vi "字符串至进制转换（个人编写）.vi"(1 "字符串":string) -> (0 "十六进制字符串":string)   [LabVIEW 2012]
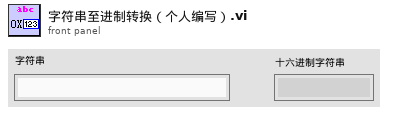
[diagram p1: front panel]
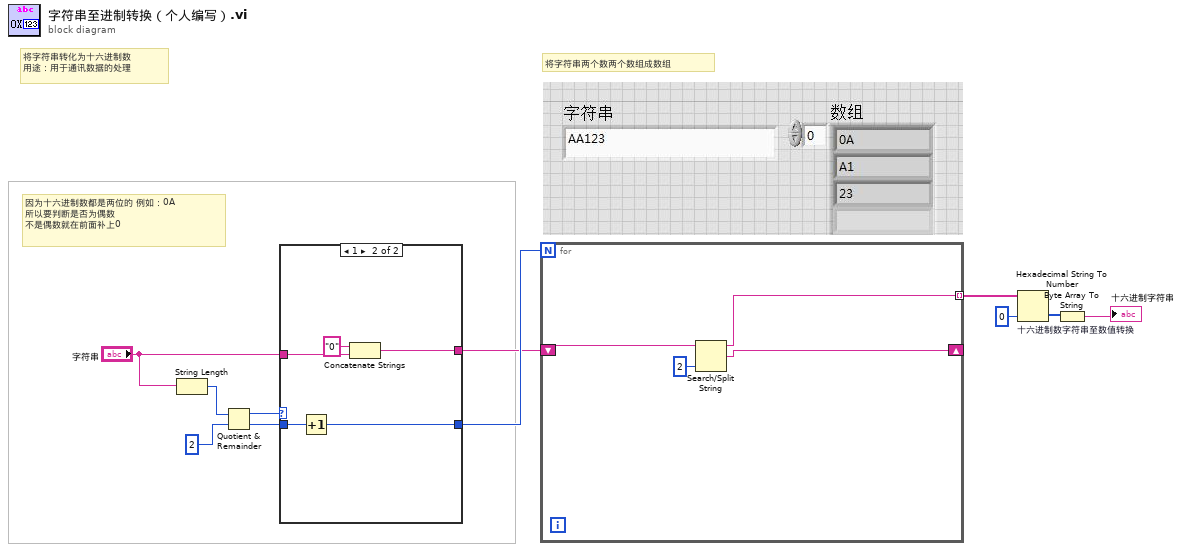
[diagram p0: block diagram]
diagram:
  # "将字符串转化为十六进制数\n用途：用于通讯数据的处理"
  # "将字符串两个数两个数组成数组"
  # "因为十六进制数都是两位的 例如：0A\n所以要判断是否为偶数\n不是偶数就在前面补上0"
  n1 = String Length(string="字符串") -> (length=w8:i32)
  n2 = Quotient & Remainder(x=w8, y=2) -> (x-y*floor(x/y)=w10:i32, floor(x/y)=w7:i32)
  n3 = case shown="1" w10 {
    tunnel: "字符串" -> [w13 w18]
    tunnel: [w13 w16] -> w5
    tunnel: w7 -> [w12 w15]
    tunnel: [w12 w14] -> w6
    frame 0, Default {
    }
    frame 1 {
      n4 = Increment(x=w15) -> (x+1=w14:i32)
      n5 = Concatenate Strings("0" ("字符串"), w18) -> (w16:string)
    }
  }
  n6 = for {
    N: w6 -> [_]
    shift-right: [w20] -> _
    shift-left: w5 -> [w22]
    tunnel: [w19] -> w4 mode=indexing
    n7 = Search/Split String(string=w22, offset (0)=2 ("偏移量(0)")) -> (substring before match=w19:string, match + rest of string=w20:string)  [unwired: 1 in, 1 out]
  }
  n8 = Hexadecimal String To Number "十六进制数字符串至数值转换"(string=w4, default (0uL)=u32 0 ("默认(0 U32)")) -> (number=w1:u32[])  [unwired: 1 in, 1 out]
  n9 = Byte Array To String(unsigned byte array=w1) -> (string=→"十六进制字符串":string)
